vi "Build Bus Controller Sequence.vi"(8 "error in (no error)":errorcluster, 11 "1553 Test in":refnum<class "1553 Test.lvclass">) -> (0 "error out":errorcluster, 3 "1553 Test out":refnum<class "1553 Test.lvclass">)   [LabVIEW 2016, in "1553 Test.lvclass"]
uses:
  1553 Test.lvclass
  Frames & Messages/Major Frame/Major Frame.lvclass
  1553 Component/1553 Component.lvclass
  Bus Controller/Bus Controller.lvclass
  Bus Controller/TypeDefs/Bus Controller Configuration.ctl
  Frames & Messages/Minor Frame/Minor Frame.lvclass
  Frames & Messages/Message/Message.lvclass
  Frames & Messages/RT-RT Message/RT-RT Message.lvclass
  Frames & Messages/TypeDefs/Command Config.ctl
  BCI-1553 API.lvlib
  Frames & Messages/TypeDefs/Message Control.ctl
  Frames & Messages/TypeDefs/Message Config.ctl
  Frames & Messages/TypeDefs/RT-RT Message Config.ctl
  1553 Board/1553 Board.lvclass
  Bus Controller/TypeDefs/Bus Controller Timeout.ctl
  Frames & Messages/TypeDefs/Command Word Count.ctl
  Frames & Messages/TypeDefs/Command SubAddress.ctl
  Frames & Messages/TypeDefs/Command Terminal Address.ctl
  Frames & Messages/TypeDefs/Command Type.ctl
  Dependencies/FPGA Interface/FPGA Interface.lvclass
  D:/R&D/cRIO 1553 2016/Windows/Frames & Messages/Message/Message.lvclass
  D:/R&D/cRIO 1553 2016/Windows/1553 SubComponent/1553 SubComponent.lvclass
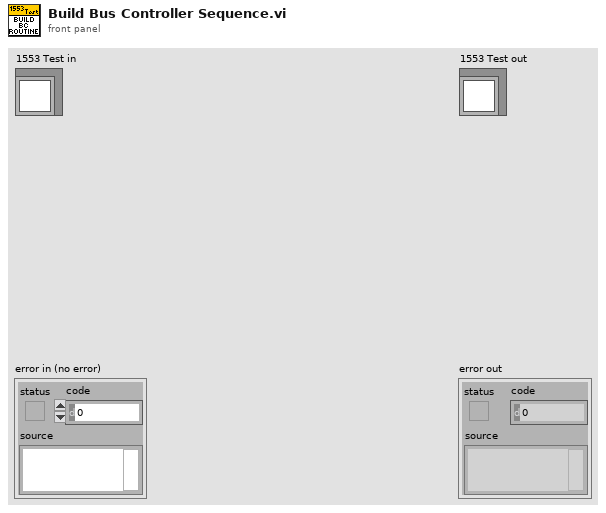
[diagram p1: front panel]
types:
  T1 = typedef "BCI-1553 API.lvlib/Message Config.ctl" = cluster{"Time to Next Msg (4 us)":u16, "Command Config":T2, "Message Control":T7}
  T2 = typedef "BCI-1553 API.lvlib/Command Config.ctl" = cluster{"Command Type":T3, "Terminal Address":T4, "SubAddress":T5, "Word Count\\Mode Code":T6, "Command Data":u16[]}
  T3 = typedef "BCI-1553 API.lvlib/Command Type.ctl" = enum16{"Transmit", "Receive"}
  T4 = typedef "BCI-1553 API.lvlib/Command Terminal Address.ctl" = enum16{"0", "1", "2", "3", "4", "5", "6", "7", "8", "9", "10", "11", "12", "13", "14", "15", "16", "17", "18", "19", "20", "21", "22", "23", "24", "25", "26", "27", "28", "29", "30", "Broadcast"}
  T5 = typedef "BCI-1553 API.lvlib/Command SubAddress.ctl" = enum16{"Mode Code", "1", "2", "3", "4", "5", "6", "7", "8", "9", "10", "11", "12", "13", "14", "15", "16", "17", "18", "19", "20", "21", "22", "23", "24", "25", "26", "27", "28", "29", "30"}
  T6 = typedef "BCI-1553 API.lvlib/Command Word Count.ctl" = enum16{"1", "2", "3", "4", "5", "6", "7", "8", "9", "10", "11", "12", "13", "14", "15", "16", "17", "18", "19", "20", "21", "22", "23", "24", "25", "26", "27", "28", "29", "30", "31", "32"}
  T7 = typedef "BCI-1553 API.lvlib/Message Control.ctl" = cluster{"MC17 Time Sync":bool, "Error Mask":bool, "Service Request Mask":bool, "Busy Mask":bool, "SubSystem Flag Mask":bool, "Terminal Flag Mask":bool, "Reserved Mask":bool, "Retry":bool, "Bus A / !Bus B":bool, "Self-Test Loopback":bool, "Broadcast Mask":bool, "EoM Interrupt":bool, "Mode Code Format":bool, "Broadcast Format":bool, "RT-RT Format":bool}
  T8 = typedef "BCI-1553 API.lvlib/RT-RT Message Config.ctl" = cluster{"Tx Command Config":T2}
  T9 = typedef "BCI-1553 API.lvlib/Bus Controller.lvclass/Bus Controller Configuration.ctl" = cluster{"Timeout":T10, "BC Retry":bool, "BC Second Retry":bool, "BC Retry Alt Bus":bool, "BC Second Retry Alt Bus":bool, "BC Retry on Status Bit":bool, "Msg Error No Data Valid":bool, "Busy Status No Data Valid":bool, "Msg Gap Timer":bool, "Watchdog Timer":bool, "Time Tag Sync":bool, "Even Time Tag Sync":bool, "Gap Check":bool, "Broadcast Mask Enable":bool}
  T10 = typedef "BCI-1553 API.lvlib/Bus Controller.lvclass/Bus Controller Timeout.ctl" = enum16{"17us", "22us", "60us", "140us"}
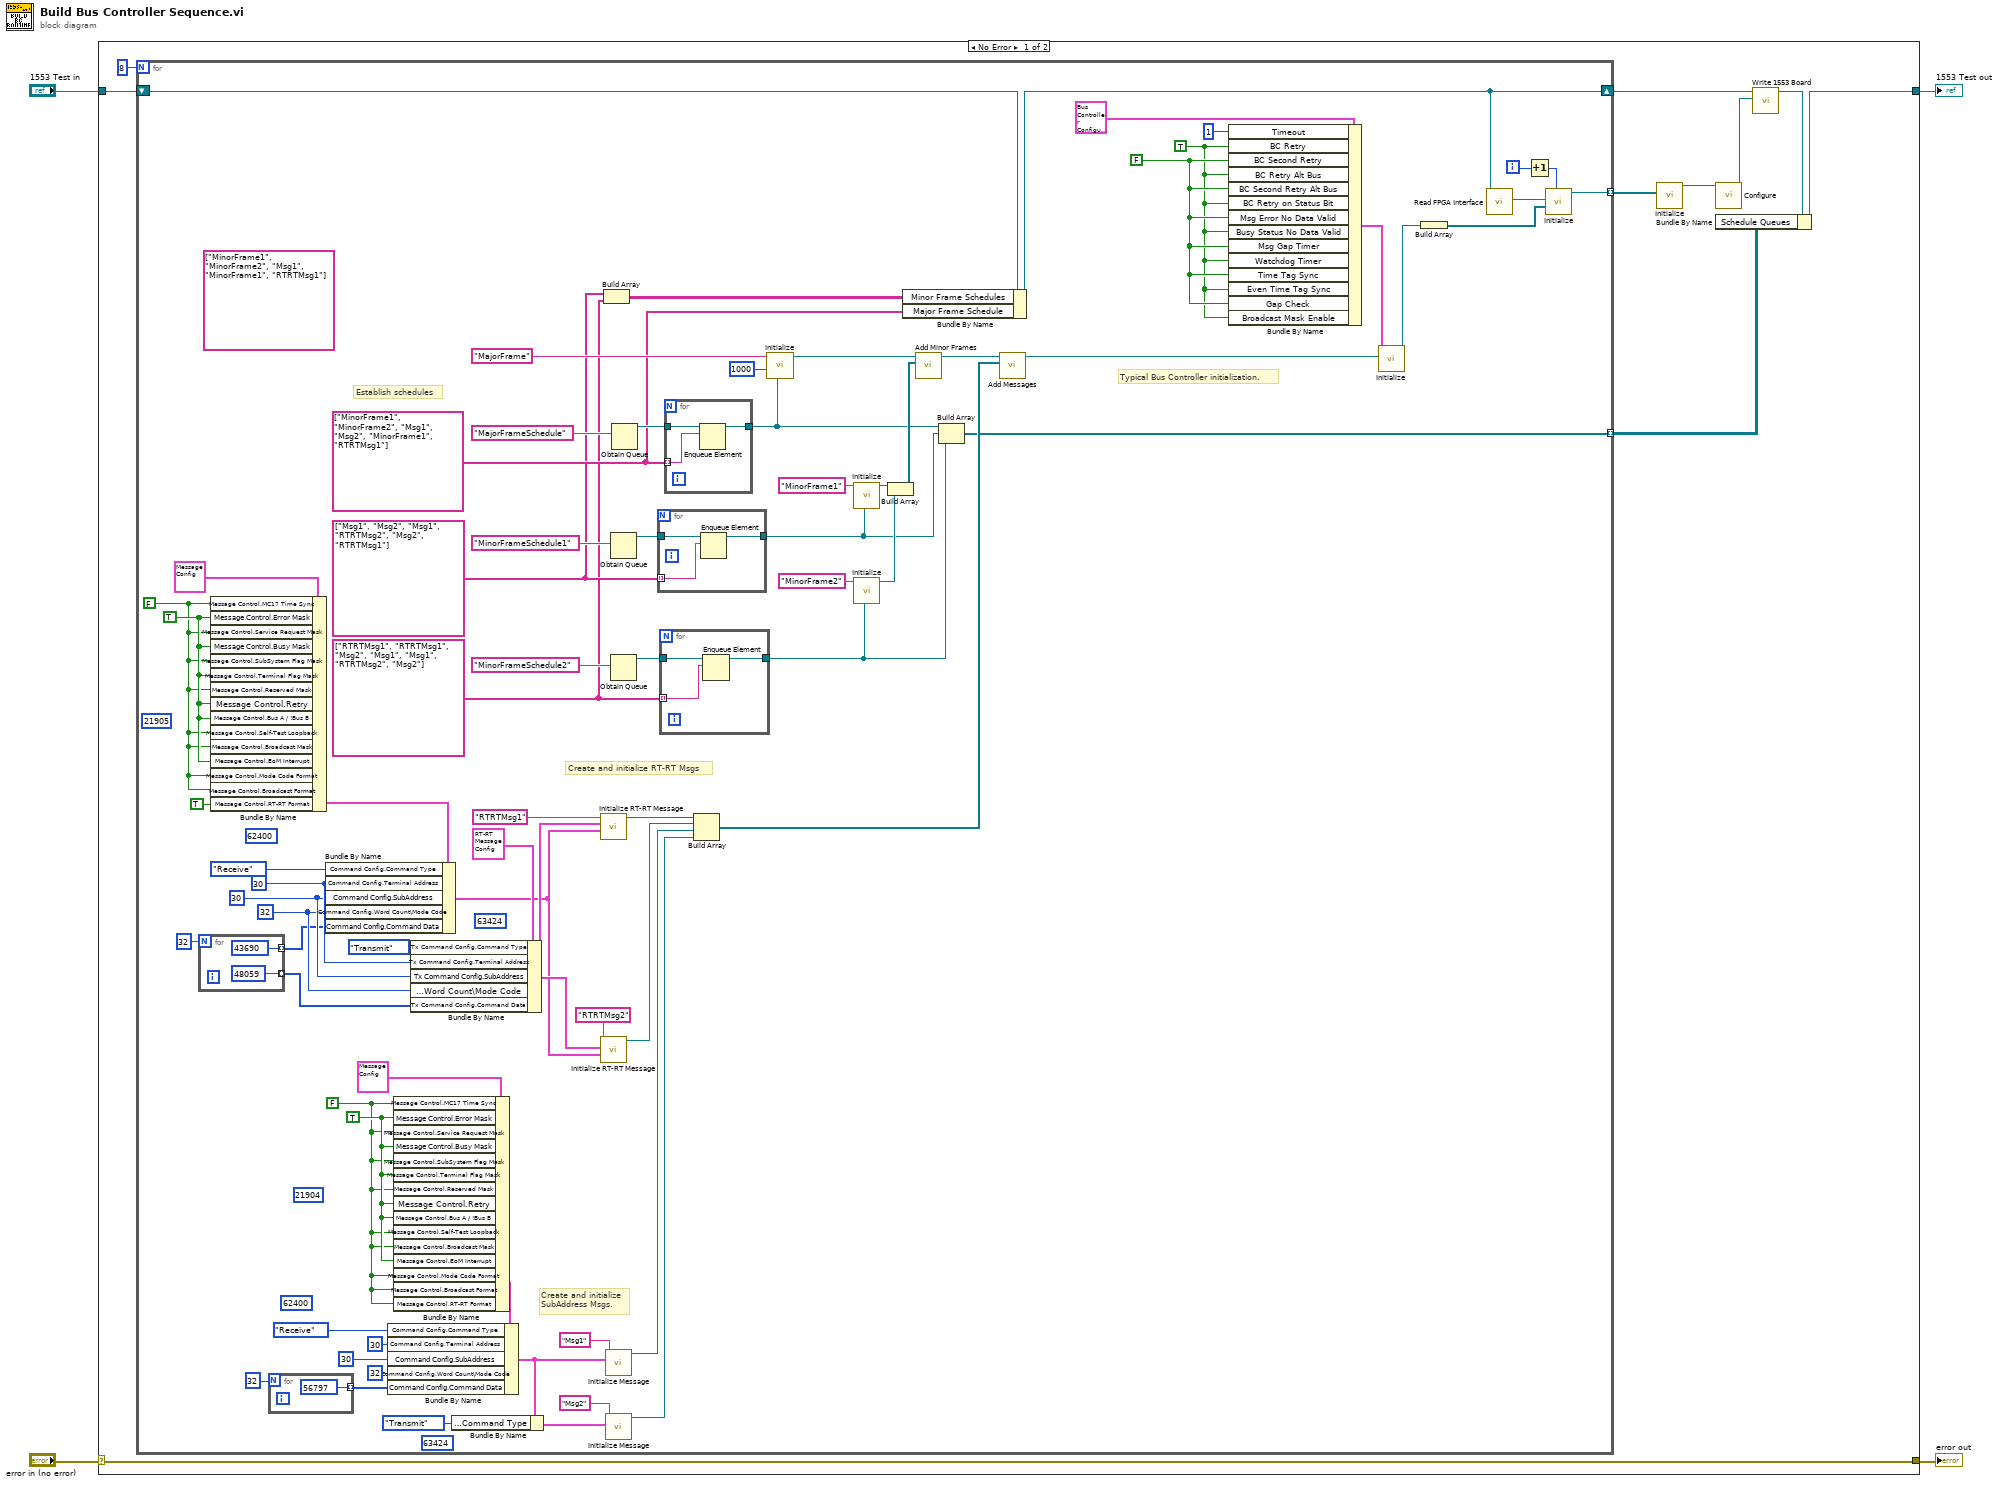
[diagram p0: block diagram]
diagram:
  n1 = case shown="No Error" "error in (no error)" {
    selector: "error in (no error)" -> [w14 w103]
    tunnel: [w14 w103] -> w3
    tunnel: [w5 w102] -> w1
    tunnel: "1553 Test in" -> [w11 w102]
    frame No Error {
      n2 = for {
        N: 8 -> [_]
        shift-right: [w31] -> w10
        shift-left: w11 -> [w32]
        tunnel: [w17] -> w8 mode=indexing
        tunnel: [w16] -> w7 mode=indexing
        i -> [w15]
        (unwired) string[] ["MinorFrame1", "MinorFrame2", "Msg1", "MinorFrame1", "RTRTMsg1"]
        (unwired) u16 63424
        (unwired) u16 62400
        (unwired) u16 63424
        (unwired) u16 62400
        (unwired) u16 21905
        (unwired) u16 21904
        w26 = string[] ["Msg1", "Msg2", "Msg1", "RTRTMsg2", "Msg2", "RTRTMsg1"]
        w25 = string[] ["RTRTMsg1", "RTRTMsg1", "Msg2", "Msg1", "Msg1", "RTRTMsg2", "Msg2"]
        w27 = string[] ["MinorFrame1", "MinorFrame2", "Msg1", "Msg2", "MinorFrame1", "RTRTMsg1"]
        w44 = TRUE ("Message Control.Error Mask")
        w43 = FALSE ("Message Control.MC17 Time Sync")
        w53 = TRUE ("Message Control.Error Mask")
        w51 = FALSE ("Message Control.MC17 Time Sync")
        w46 = u16 32 ("Command Config.WC/MC (1-32)")
        w47 = u16 30 ("Command Config.SubAddress (1-30)")
        w48 = u16 30 ("Command Config.Terminal Address (0-30)")
        w81 = FALSE ("BC Second Retry")
        w80 = TRUE ("BC Retry")
        # "Create and initialize\nSubAddress Msgs."
        # "Create and initialize RT-RT Msgs"
        # "Establish schedules"
        # "Typical Bus Controller initialization."
        n3 = for {
          N: 32 -> [_]
          tunnel: [u16 43690] -> w23 mode=indexing
          tunnel: [u16 48059] -> w22 mode=indexing
        }
        n4 = Bundle By Name(cluster=T1 {"Time to Next Msg (4 us)"=100, "Command Config"={"Command Type"=enum."Transmit", "Terminal Address"=enum."0", "SubAddress"=enum."Mode Code", "Word Count\\Mode Code"=enum."1", "Command Data"=[]}, "Message Control"={"MC17 Time Sync"=FALSE, "Error Mask"=FALSE, "Service Request Mask"=FALSE, "Busy Mask"=FALSE, "SubSystem Flag Mask"=FALSE, "Terminal Flag Mask"=FALSE, "Reserved Mask"=FALSE, "Retry"=FALSE, "Bus A / !Bus B"=FALSE, "Self-Test Loopback"=FALSE, "Broadcast Mask"=FALSE, "EoM Interrupt"=FALSE, "Mode Code Format"=FALSE, "Broadcast Format"=FALSE, "RT-RT Format"=FALSE}} ("Message Config"), "Message Control.MC17 Time Sync"=w51, "Message Control.Error Mask"=w53, "Message Control.Service Request Mask"=w51, "Message Control.Busy Mask"=w53, "Message Control.SubSystem Flag Mask"=w51, "Message Control.Terminal Flag Mask"=w53, "Message Control.Reserved Mask"=w51, "Message Control.Retry"=w53, "Message Control.Bus A / !Bus B"=w53, "Message Control.Self-Test Loopback"=w51, "Message Control.Broadcast Mask"=w51, "Message Control.EoM Interrupt"=w53, "Message Control.Mode Code Format"=w51, "Message Control.Broadcast Format"=w51, "Message Control.RT-RT Format"=TRUE) -> (w54:T1)
        n5 = for {
          N: 32 -> [_]
          tunnel: [u16 56797] -> w36 mode=indexing
        }
        n6 = Bundle By Name(cluster=w54, "Command Config.Command Type"=enum16{"Transmit", "Receive"}."Receive", "Command Config.Terminal Address"=w48, "Command Config.SubAddress"=w47, "Command Config.Word Count\\Mode Code"=w46, "Command Config.Command Data"=w23) -> (w20:T1)
        n7 = Bundle By Name(cluster=T1 {"Time to Next Msg (4 us)"=100, "Command Config"={"Command Type"=enum."Transmit", "Terminal Address"=enum."0", "SubAddress"=enum."Mode Code", "Word Count\\Mode Code"=enum."1", "Command Data"=[]}, "Message Control"={"MC17 Time Sync"=FALSE, "Error Mask"=FALSE, "Service Request Mask"=FALSE, "Busy Mask"=FALSE, "SubSystem Flag Mask"=FALSE, "Terminal Flag Mask"=FALSE, "Reserved Mask"=FALSE, "Retry"=FALSE, "Bus A / !Bus B"=FALSE, "Self-Test Loopback"=FALSE, "Broadcast Mask"=FALSE, "EoM Interrupt"=FALSE, "Mode Code Format"=FALSE, "Broadcast Format"=FALSE, "RT-RT Format"=FALSE}} ("Message Config"), "Message Control.MC17 Time Sync"=w43, "Message Control.Error Mask"=w44, "Message Control.Service Request Mask"=w43, "Message Control.Busy Mask"=w44, "Message Control.SubSystem Flag Mask"=w43, "Message Control.Terminal Flag Mask"=w44, "Message Control.Reserved Mask"=w43, "Message Control.Retry"=w44, "Message Control.Bus A / !Bus B"=w44, "Message Control.Self-Test Loopback"=w43, "Message Control.Broadcast Mask"=w43, "Message Control.EoM Interrupt"=w44, "Message Control.Mode Code Format"=w43, "Message Control.Broadcast Format"=w43, "Message Control.RT-RT Format"=w43) -> (w41:T1)
        n8 = Bundle By Name(cluster=w41, "Command Config.Command Type"=enum16{"Transmit", "Receive"}."Receive", "Command Config.Terminal Address"=u16 30 ("Command Config.Terminal Address (0-30)"), "Command Config.SubAddress"=u16 30 ("Command Config.SubAddress (1-30)"), "Command Config.Word Count\\Mode Code"=u16 32 ("Command Config.WC/MC (1-32)"), "Command Config.Command Data"=w36) -> (w34:T1)
        n9 = Bundle By Name(cluster=T8 {"Tx Command Config"={"Command Type"=enum."Transmit", "Terminal Address"=enum."0", "SubAddress"=enum."Mode Code", "Word Count\\Mode Code"=enum."1", "Command Data"=[]}} ("RT-RT Message Config"), "Tx Command Config.Command Type"=enum16{"Transmit", "Receive"}."Transmit", "Tx Command Config.Terminal Address"=w48, "Tx Command Config.SubAddress"=w47, "Tx Command Config.Word Count\\Mode Code"=w46, "Tx Command Config.Command Data"=w22) -> (w21:T8)
        n10 = Bundle By Name(cluster=w34, "Command Config.Command Type"=enum16{"Transmit", "Receive"}."Transmit") -> (w33:T1)
        n11 = call "Initialize RT-RT Message.vi"("Receive Message Config"=w20, "Transmit Message Config"=w21, "ID"="RTRTMsg1") -> ("RT-RT Message out"=w63:refnum<class "RT-RT Message.lvclass">)  [unwired: 7 in, 1 out]
        n12 = call "Initialize RT-RT Message.vi"("Receive Message Config"=w20, "Transmit Message Config"=w21, "ID"="RTRTMsg2") -> ("RT-RT Message out"=w58:refnum<class "RT-RT Message.lvclass">)  [unwired: 7 in, 1 out]
        n13 = Build Array(w26, w25) -> (w24:string[][])
        n14 = call "Initialize Message.vi"("Message  Config"=w34, "ID"="Msg1") -> ("Message out"=w59:refnum<class "Message.lvclass">)  [unwired: 8 in, 1 out]
        n15 = call "Initialize Message.vi"("Message  Config"=w33, "ID"="Msg2") -> ("Message out"=w62:refnum<class "Message.lvclass">)  [unwired: 8 in, 1 out]
        n16 = Obtain Queue(element data type="MinorFrameSchedule1") -> (queue out=w75:refnum<queue>)  [unwired: 4 in, 2 out]
        n17 = Obtain Queue(element data type="MinorFrameSchedule2") -> (queue out=w74:refnum<queue>)  [unwired: 4 in, 2 out]
        n18 = Obtain Queue(element data type="MajorFrameSchedule") -> (queue out=w79:refnum<queue>)  [unwired: 4 in, 2 out]
        n19 = for {
          tunnel: w75 -> [w98]
          tunnel: [w97] -> w29
          tunnel: w26 -> [w96] mode=indexing
          n20 = Enqueue Element(queue=w98, element=w96) -> (queue out=w97:refnum<queue>)  [unwired: 2 in, 2 out]
        }
        n21 = for {
          tunnel: w74 -> [w95]
          tunnel: [w94] -> w28
          tunnel: w25 -> [w93] mode=indexing
          n22 = Enqueue Element(queue=w95, element=w93) -> (queue out=w94:refnum<queue>)  [unwired: 2 in, 2 out]
        }
        n23 = for {
          tunnel: w79 -> [w101]
          tunnel: [w100] -> w30
          tunnel: w27 -> [w99] mode=indexing
          n24 = Enqueue Element(queue=w101, element=w99) -> (queue out=w100:refnum<queue>)  [unwired: 2 in, 2 out]
        }
        n25 = Build Array(w63, w58, w59, w62) -> (w61:refnum<class "Message.lvclass">[])
        n26 = call "Initialize.vi"("Schedule"=w30, "Minor Frame Time (100 us)"=u16 1000 ("Minor Frame Time (us)"), "ID"="MajorFrame") -> ("Major Frame out"=w78:refnum<class "Major Frame.lvclass">)  [unwired: 7 in, 1 out]
        n27 = call "Initialize.vi"("Schedule"=w29, "ID"="MinorFrame1") -> ("Minor Frame out"=w71:refnum<class "Minor Frame.lvclass">)  [unwired: 8 in, 1 out]
        n28 = call "Initialize.vi"("Schedule"=w28, "ID"="MinorFrame2") -> ("Minor Frame out"=w70:refnum<class "Minor Frame.lvclass">)  [unwired: 8 in, 1 out]
        n29 = Build Array(w71, w70) -> (w69:refnum<class "Minor Frame.lvclass">[])
        n30 = Bundle By Name(cluster=w32, "Minor Frame Schedules"=w24, "Major Frame Schedule"=w27) -> (w31:refnum<class "1553 Test.lvclass">)
        n31 = call-dynamic "Add Minor Frames.vi"("Minor Frames"=w69, "Major Frame in"=w78) -> ("Major Frame out"=w68:refnum<class "Major Frame.lvclass">)  [unwired: 8 in, 1 out]
        n32 = Build Array(w30, w29, w28) -> (w16:refnum<queue>[])
        n33 = call-dynamic "Add Messages.vi"("Messages"=w61, "Major Frame in"=w68) -> ("Major Frame out"=w60:refnum<class "Major Frame.lvclass">)  [unwired: 8 in, 1 out]
        n34 = Bundle By Name(cluster=T9 {"Timeout"=enum."17us", "BC Retry"=FALSE, "BC Second Retry"=FALSE, "BC Retry Alt Bus"=FALSE, "BC Second Retry Alt Bus"=FALSE, "BC Retry on Status Bit"=FALSE, "Msg Error No Data Valid"=FALSE, "Busy Status No Data Valid"=FALSE, "Msg Gap Timer"=FALSE, "Watchdog Timer"=FALSE, "Time Tag Sync"=FALSE, "Even Time Tag Sync"=FALSE, "Gap Check"=FALSE, "Broadcast Mask Enable"=FALSE} ("Configuration"), "Timeout"=u16 1 ("BC Timeout"), "BC Retry"=w80, "BC Second Retry"=w81, "BC Retry Alt Bus"=w80, "BC Second Retry Alt Bus"=w81, "BC Retry on Status Bit"=w80, "Msg Error No Data Valid"=w81, "Busy Status No Data Valid"=w80, "Msg Gap Timer"=w81, "Watchdog Timer"=w80, "Time Tag Sync"=w81, "Even Time Tag Sync"=w80, "Gap Check"=w81, "Broadcast Mask Enable"=w80) -> (w83:T9)
        n35 = call "Initialize.vi"("Major Frame"=w60, "Configuration"=w83) -> ("Bus Controller out"=w86:refnum<class "Bus Controller.lvclass">)  [unwired: 8 in, 1 out]
        n36 = Build Array(w86) -> (w85:refnum<class "Bus Controller.lvclass">[])
        n37 = call-dynamic "Read FPGA Interface.vi"("1553 Test in"=w31) -> ("FPGA Interface"=w19:refnum<class "FPGA Interface.lvclass">)  [unwired: 8 in, 2 out]
        n38 = Increment(x=w15) -> (x+1=w18:i32)
        n39 = call "Initialize.vi"("Component ID (1-8)"=w18, "SubComponents"=w85, "FPGA Interface"=w19) -> ("1553 Component out"=w17:refnum<class "1553 Component.lvclass">)  [unwired: 7 in, 1 out]
      }
      n40 = call "Initialize.vi"("Components"=w8) -> ("1553 Board out"=w13:refnum<class "1553 Board.lvclass">)  [unwired: 9 in, 1 out]
      n41 = call-dynamic "Configure.vi"("1553 Board in"=w13) -> ("1553 Board out"=w12:refnum<class "1553 Board.lvclass">)  [unwired: 9 in, 1 out]
      n42 = call-dynamic "Write 1553 Board.vi"("1553 Board"=w12, "1553 Test in"=w10) -> ("1553 Test out"=w6:refnum<class "1553 Test.lvclass">)  [unwired: 8 in, 1 out]
      n43 = Bundle By Name(cluster=w6, "Schedule Queues"=w7) -> (w5:refnum<class "1553 Test.lvclass">)
    }
    frame Error {
    }
  }
  "error out" <- w3
  "1553 Test out" <- w1
